vi "9375 DIO FPGA.vi"() -> ()   [LabVIEW 2023]
uses:
  <vilib>/eio/EIONode/EIONode.xnode
  <vilib>/rvi/eio/common/nirviEmuTemplateMethod_errors.vi
panel:
  out "DI 7:0":bool[](array[boolean])
  in  "DO 7:0":bool[](array[boolean])=[FALSE, FALSE, FALSE, FALSE, FALSE, FALSE, FALSE, FALSE]
  in  "DO 15:8":bool[](array[boolean])=[FALSE, FALSE, FALSE, FALSE, FALSE, FALSE, FALSE, FALSE]
  in  "stop":bool
  out "DI 15:8":bool[](array[boolean])
  out "FPGA Error Out":errorcluster
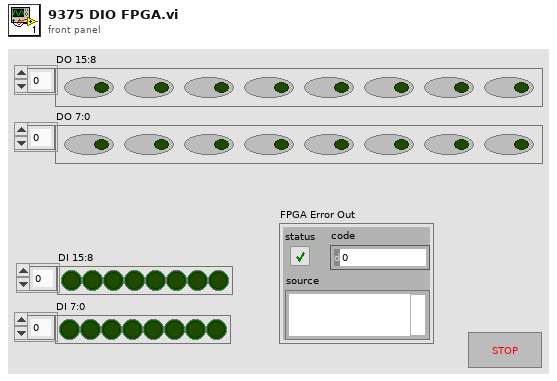
[diagram p1: front panel]
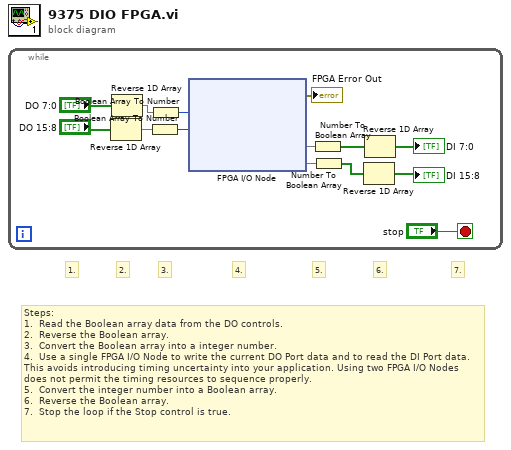
[diagram p0: block diagram]
diagram:
  # "5."
  # "6."
  # "Steps: \n1.  Read the Boolean array data from the DO controls.\n2.  Reverse the Boolean array.\n3.  Convert the Boolean array into a integer number.\n4.  Use a single FPGA I/O Node to write the current DO Port data and to read the DI Port data. This avoids introducing timing uncertainty into your application. Using two FPGA I/O Nodes does not permit the timing resources to sequence properly.\n5.  Convert the integer number into a Boolean array.\n6.  Reverse the Boolean array. \n7.  Stop the loop if the Stop control is true."
  # "7."
  # "4."
  # "3."
  # "2."
  # "1."
  n1 = while {
    stop <- "stop" stop-if-true
    n2 = Reverse 1D Array(array="DO 15:8") -> (reversed array=w11:bool[])
    n3 = Reverse 1D Array(array="DO 7:0") -> (reversed array=w12:bool[])
    n4 = Boolean Array To Number(Boolean array=w11) -> (number=w9:u8)
    n5 = Boolean Array To Number(Boolean array=w12) -> (number=w10:u8)
    n6 = xnode "FPGA I/O Node"("Mod1/DO7:0"=w10, "Mod1/DO15:8"=w9) -> ("error out"=→"FPGA Error Out":errorcluster, "Mod1/DI7:0"=w14, "Mod1/DI15:8"=w13)  [unwired: 5 in, 4 out]
    n7 = Number To Boolean Array(number=w14) -> (Boolean array=w7:bool[])
    n8 = Number To Boolean Array(number=w13) -> (Boolean array=w8:bool[])
    n9 = Reverse 1D Array(array=w8) -> (reversed array=→"DI 15:8":bool[])
    n10 = Reverse 1D Array(array=w7) -> (reversed array=→"DI 7:0":bool[])
  }
